vi "流量计.vi"() -> ()   [LabVIEW 2016, in "流量计集成.lvlib"]
uses:
  <vilib>/Plasmionique/MB Master/MB_Master_Serial/MB_Master_Serial.lvclass
  D:/Program Files (x86)/National Instruments/LabVIEW 2016/vi.lib/Plasmionique/MB Master/MB_Master/MB_Master.lvclass
  <vilib>/Analysis/baseanly.llb/Mean (DBL).vi
  <vilib>/Utility/config.llb/NI_LVConfig.lvlib
  <vilib>/Analysis/NI_AALBase.lvlib
panel:
  in  "运行模式":enum16{"按周期模式", "全常规模式"}(ring)=enum."全常规模式"
  in  "流量计启用 5":bool
  in  "数量 5":u16
  out "流量计类型 5":T1=enum."WL1A1明渠流量计"
  in  "流量计启用 4":bool
  in  "数量 4":u16
  out "流量计类型 4":T1=enum."博意达流量计"
  out "平均水位":dbl
  out "总累积流量":dbl
  out "平均流速":dbl
  out "总流量":dbl
  in  "选项卡控件":T2(tab)
  out "数组":T3[](array[typedef])
  out "数组 2":T4[](array[typedef]) {"累积流量单位" items=["L", "M3", "T", "USG"]; "瞬时流量单位" items=["L/S", "L/M", "L/H", "M3/S", "M3/M", "M3/H", "T/S", "T/M", "T/H", "GPS", "GPM", "GPH"]}
  out "数组 3":T7[](array[typedef])
  out "数组 4":T3[](array[typedef])
  out "数组 5":T3[](array[typedef])
  out "MB_Serial session":refnum<class "MB_Master_Serial.lvclass">
  in  "斯坦道功率测流":bool
  in  "流量计启用 3":bool
  in  "数量 3":u16
  out "流量计类型 3":T1=enum."斯坦道功率测流"
  in  "流量计启用 2":bool
  in  "数量 2":u16
  out "流量计类型 2":T1=enum."MGG/KL QC"
  in  "数量":u16
  out "流量计类型":T1
  in  "流量计启用":bool
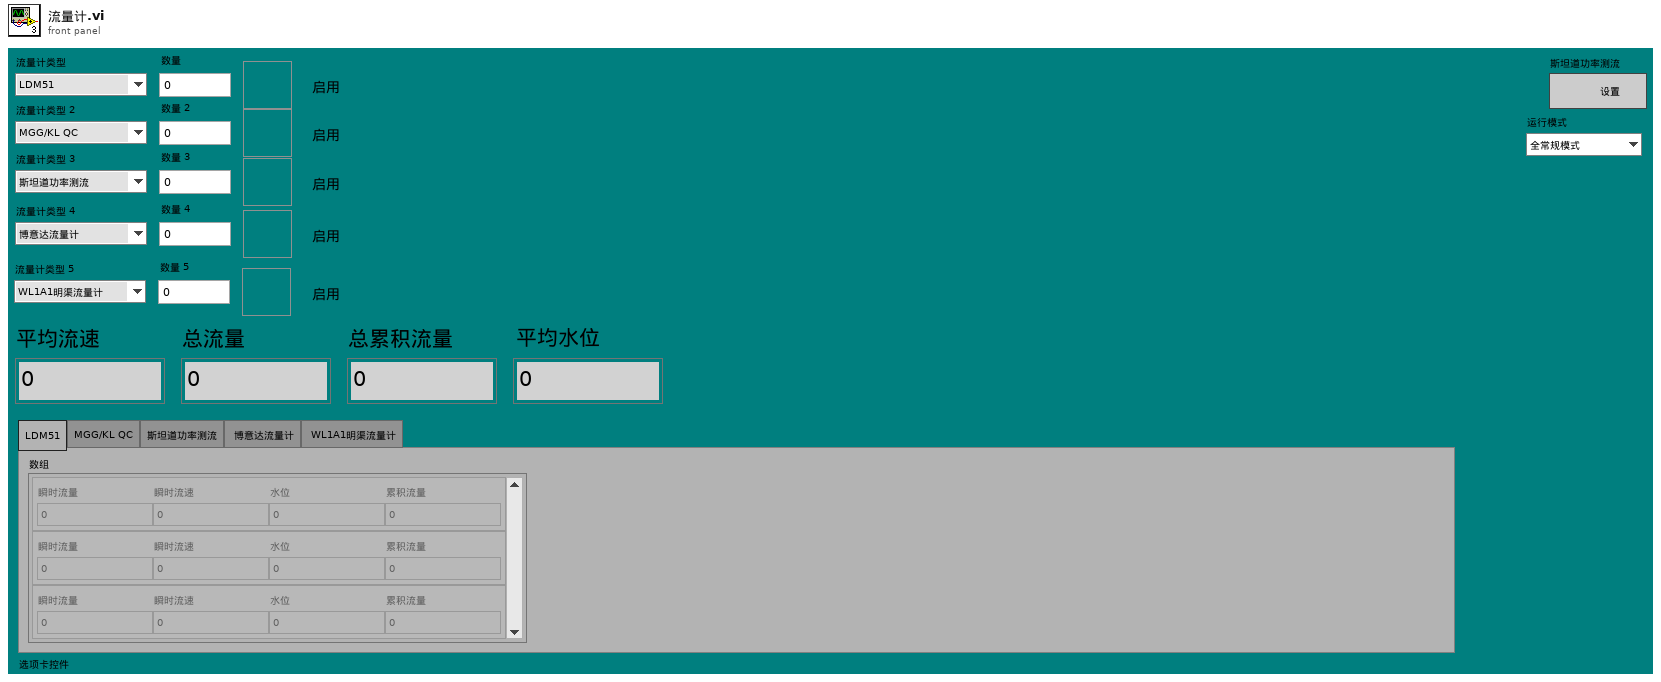
[diagram p1: front panel]
types:
  T1 = typedef "流量计集成.lvlib/流量计类型.ctl" = enum16{"LDM51", "MGG/KL QC", "斯坦道功率测流", "博意达流量计", "SL1500-3G", "WL1A1明渠流量计"}
  T2 = enum32{"LDM51", "MGG/KL QC", "斯坦道功率测流", " 博意达流量计", " WL1A1明渠流量计"}
  T3 = typedef "流量计集成.lvlib/LDM51明渠流量计.lvlib/读取值.ctl" = cluster{"瞬时流量":sgl, "瞬时流速":sgl, "水位":sgl, "累积流量":sgl}
  T4 = typedef "流量计集成.lvlib/MGG-KL-QC流量计.lvlib/读取值.ctl" = cluster{"瞬时流量":sgl, "瞬时流速":sgl, "流量百分比":sgl, "流体电导比":sgl, "正向累积数值":sgl, "反向累积数值":sgl, "瞬时流量单位":T5, "累积流量单位":T6, "上限报警":u16, "下限报警":u16, "空管报警":u16, "系统报警":u16}
  T5 = typedef "流量计集成.lvlib/MGG-KL-QC流量计.lvlib/瞬时流量单位.ctl" = u16
  T6 = typedef "流量计集成.lvlib/MGG-KL-QC流量计.lvlib/累积流量单位.ctl" = u16
  T7 = typedef "流量计集成.lvlib/斯坦道功率测流.lvlib/状态值.ctl" = cluster{"1号瞬时流量":dbl, "2号瞬时流量":dbl, "3号瞬时流量":dbl, "4号瞬时流量":dbl, "5号瞬时流量":dbl, "6号瞬时流量":dbl, "1号累积流量":dbl, "2号累积流量":dbl, "3号累积流量":dbl, "4号累积流量":dbl, "5号累积流量":dbl, "6号累积流量":dbl, "总瞬时流量":dbl, "总累积流量":dbl}
  T8 = cluster{"时间标识":timestamp, "测量模式":string, "数据类型":string, "监测值":sgl, "单位":string, "数据标识":string, "因子编码":string}
  T9 = typedef "LVDateTimeRec.ctl" = cluster{"秒数的小数部分":dbl, "秒":i32, "分":i32, "时":i32, "日":i32, "月":i32, "年":i32, "天数（周）":i32, "天数（年）":i32, "DST":i32}
  T10 = typedef "流量计集成.lvlib/博意达流量计.lvlib/读取值.ctl" = cluster{"瞬时流量":sgl, "瞬时流速":sgl, "水位":sgl, "累积流量":sgl}
  T11 = typedef "NI_LVConfig.lvlib/Config Data RefNum.ctl" = refnum<k1>
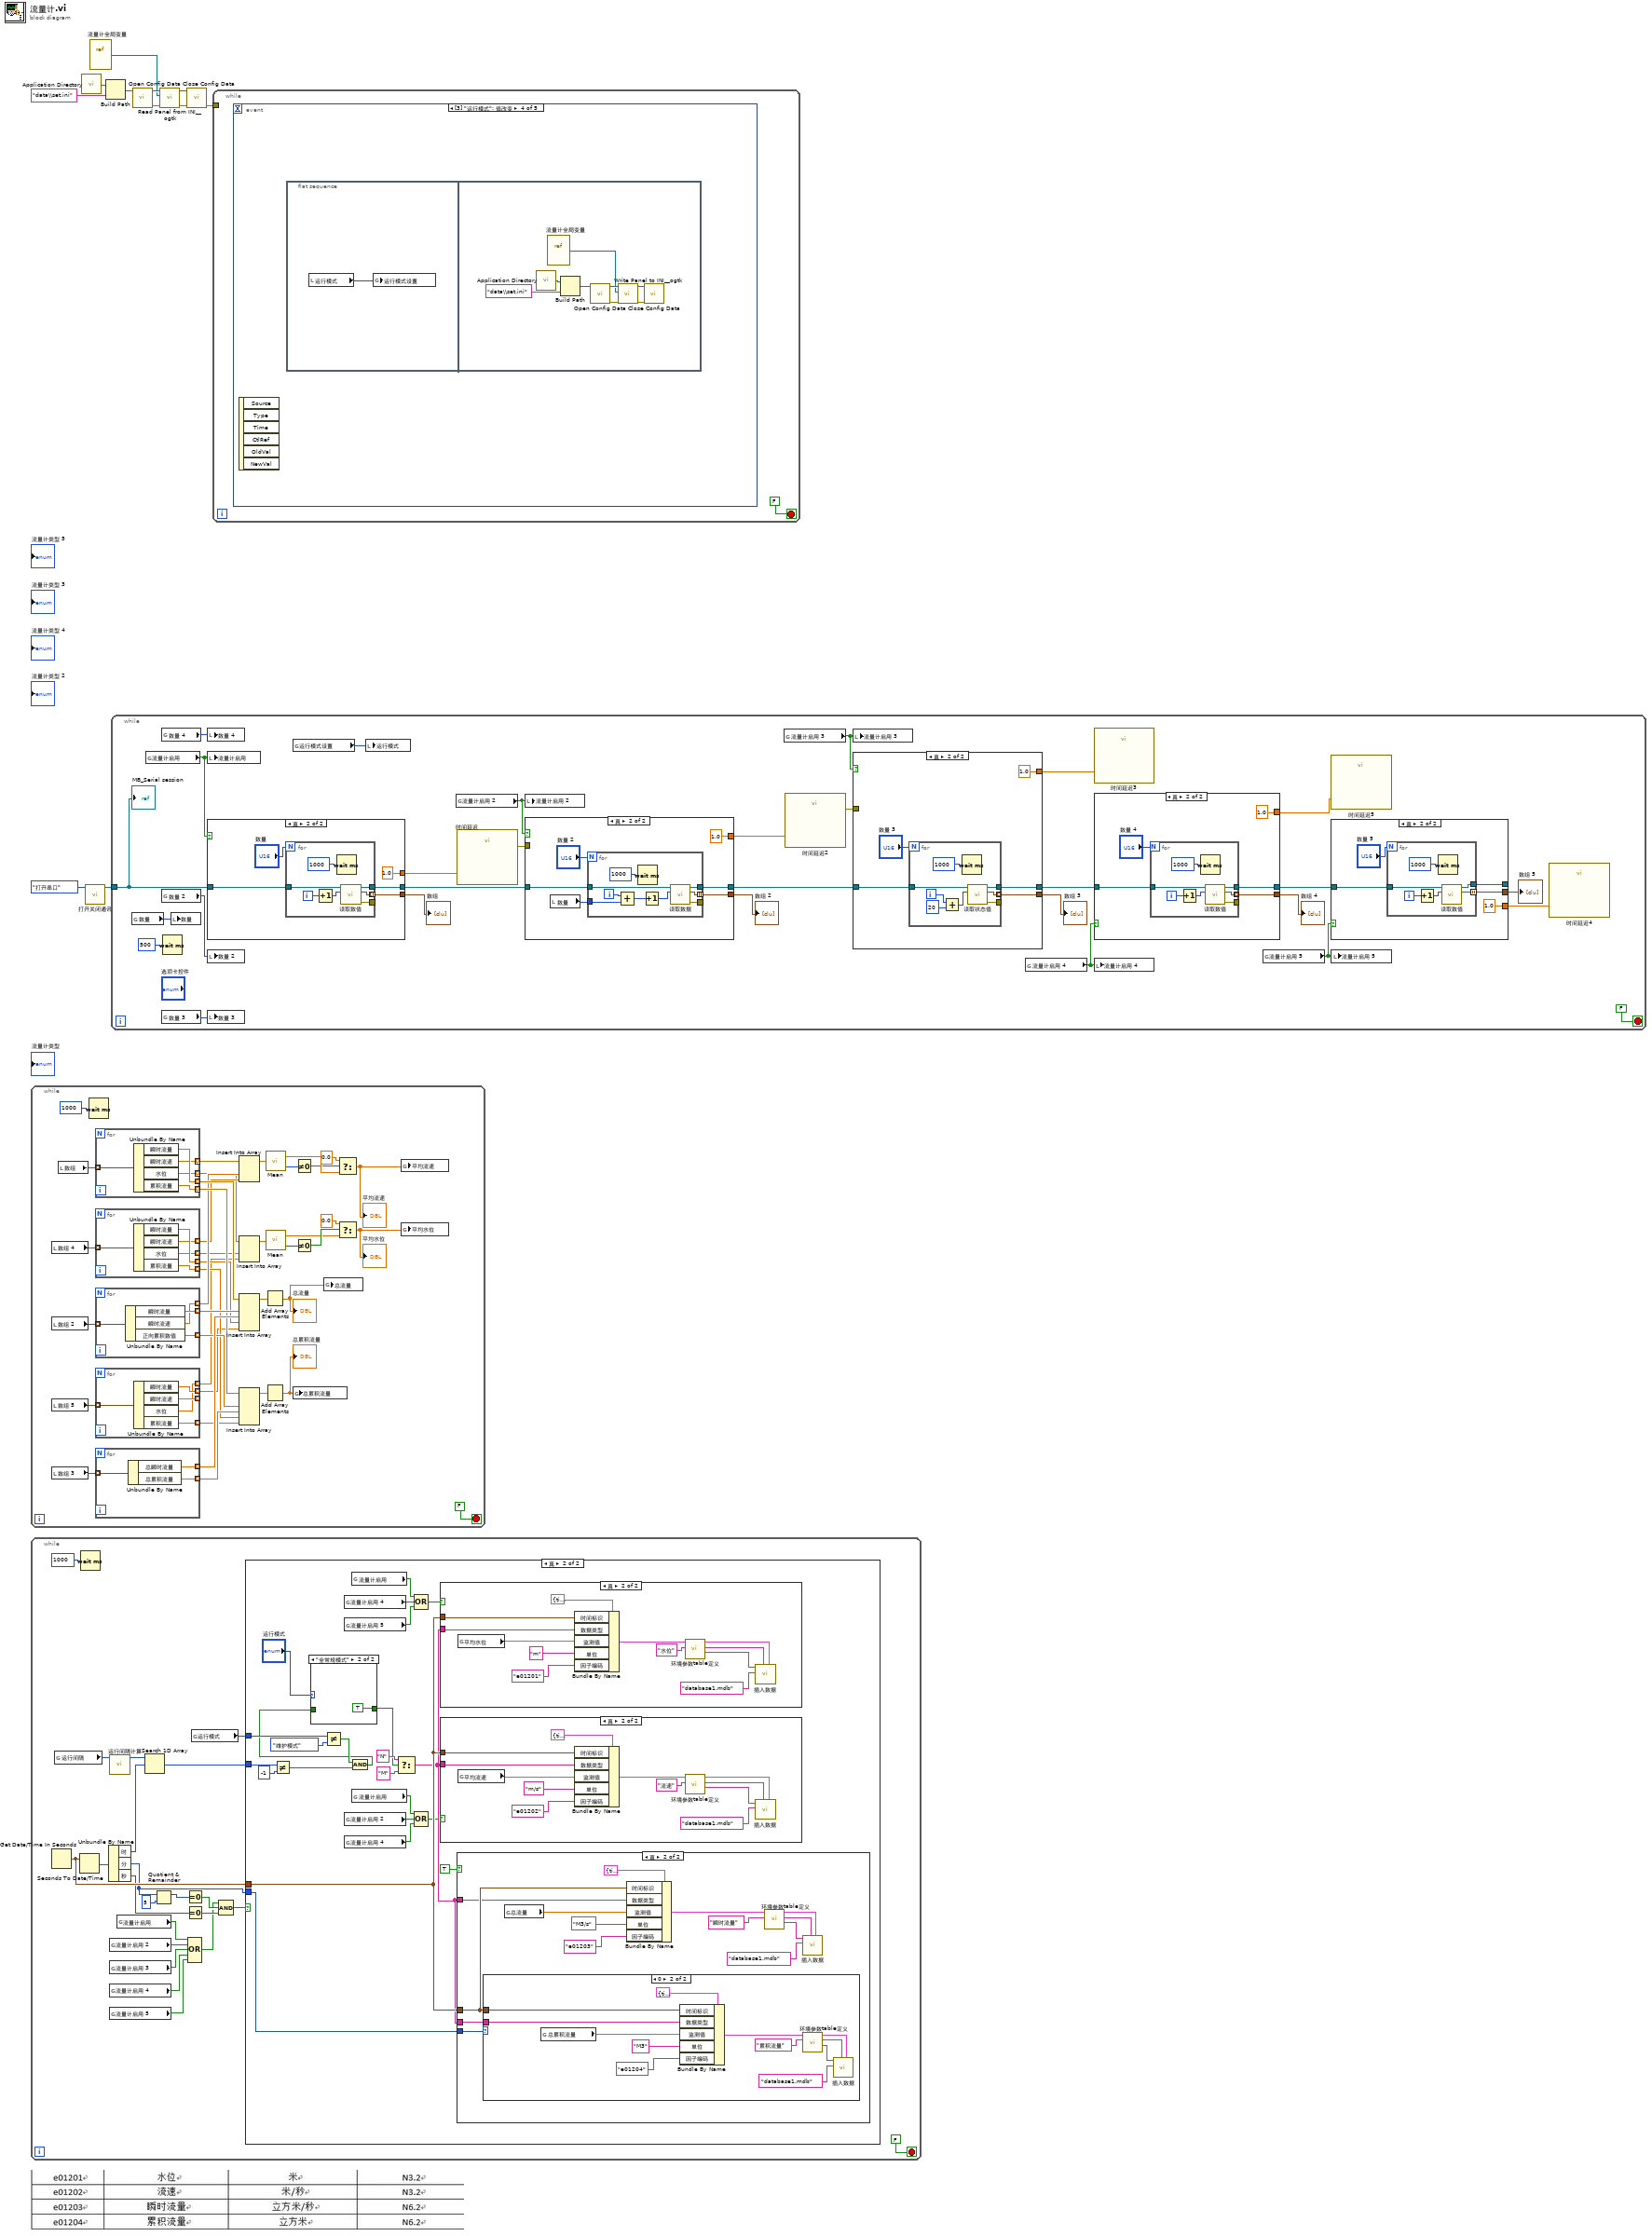
[diagram p0: block diagram]
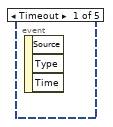
[diagram p8: hidden frame]
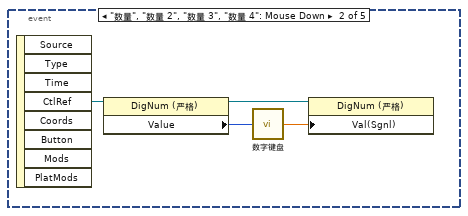
[diagram p9: hidden frame]
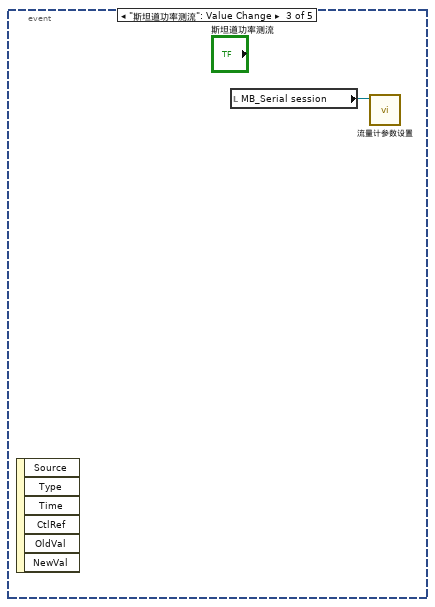
[diagram p10: hidden frame]
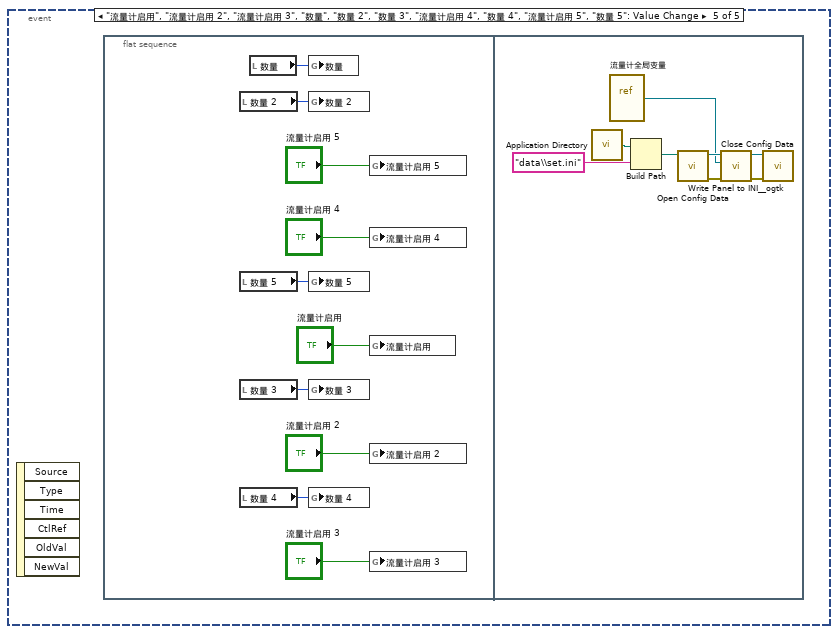
[diagram p11: hidden frame]
diagram:
  n1 = while {
    stop <- FALSE stop-if-true
    n2 = local read "数组 4"() -> (w22:T3[])
    n3 = local read "数组 2"() -> (w47:T4[])
    n4 = local read "数组 5"() -> (w15:T3[])
    n5 = local read "数组 3"() -> (w46:T7[])
    n6 = local read "数组"() -> (w50:T3[])
    n7 = Wait (ms)(milliseconds to wait=u32 1000 ("等待时间（毫秒）")) -> ()  [unwired: 1 out]
    n8 = for {
      tunnel: w50 -> [w72] mode=indexing
      tunnel: [w71] -> w45 mode=indexing
      tunnel: [w70] -> w37 mode=indexing
      tunnel: [w69] -> w19 mode=indexing
      tunnel: [w68] -> w42 mode=indexing
      n9 = Unbundle By Name(w72) -> ("瞬时流量"=w71:sgl, "瞬时流速"=w70:sgl, "水位"=w69:sgl, "累积流量"=w68:sgl)
    }
    n10 = for {
      tunnel: w22 -> [w60] mode=indexing
      tunnel: [w59] -> w20 mode=indexing
      tunnel: [w58] -> w21 mode=indexing
      tunnel: [w57] -> w17 mode=indexing
      tunnel: [w56] -> w16 mode=indexing
      n11 = Unbundle By Name(w60) -> ("瞬时流量"=w59:sgl, "瞬时流速"=w58:sgl, "水位"=w57:sgl, "累积流量"=w56:sgl)
    }
    n12 = for {
      tunnel: w47 -> [w67] mode=indexing
      tunnel: [w66] -> w44 mode=indexing
      tunnel: [w65] -> w36 mode=indexing
      tunnel: [w64] -> w41 mode=indexing
      n13 = Unbundle By Name(w67) -> ("瞬时流量"=w66:sgl, "瞬时流速"=w65:sgl, "正向累积数值"=w64:sgl)
    }
    n14 = for {
      tunnel: w15 -> [w55] mode=indexing
      tunnel: [w54] -> w13 mode=indexing
      tunnel: [w53] -> _ mode=indexing
      tunnel: [w52] -> w12 mode=indexing
      tunnel: [w51] -> w14 mode=indexing
      n15 = Unbundle By Name(w55) -> ("瞬时流量"=w54:sgl, "瞬时流速"=w53:sgl, "水位"=w52:sgl, "累积流量"=w51:sgl)
    }
    n16 = for {
      tunnel: w46 -> [w63] mode=indexing
      tunnel: [w62] -> w43 mode=indexing
      tunnel: [w61] -> w40 mode=indexing
      n17 = Unbundle By Name(w63) -> ("总瞬时流量"=w62:dbl, "总累积流量"=w61:dbl)
    }
    n18 = Insert Into Array(array=w37, new element #1=w36, new element #2=w21) -> (w31:sgl[])  [unwired: 1 in]
    n19 = Insert Into Array(array=w19, new element #1=w17, new element #2=w12) -> (w18:sgl[])  [unwired: 1 in]
    n20 = Insert Into Array(array=w45, new element #1=w44, new element #2=w43, new element #3=w20, new element #4=w13) -> (w39:sgl[])  [unwired: 1 in]
    n21 = Insert Into Array(array=w42, new element #1=w41, new element #2=w40, new element #3=w16, new element #4=w14) -> (w38:sgl[])  [unwired: 1 in]
    n22 = Add Array Elements(numeric array=w39) -> (sum=w26:sgl)
    "总流量" <- w26
    n23 = Add Array Elements(numeric array=w38) -> (sum=w24:sgl)
    "总累积流量" <- w24
    n24 = call-poly <vilib>:"Mean.vi"("X"=w31) -> ("mean"=w35:dbl, "error"=w32:i32)
    n25 = call-poly <vilib>:"Mean.vi"("X"=w18) -> ("mean"=w27:dbl, "error"=w30:i32)
    n26 = global write "流量计全局变量.vi" "总累积流量"(w24) -> ()
    n27 = Not Equal To 0?(x=w32) -> (x != 0?=w33:bool)
    n28 = Not Equal To 0?(x=w30) -> (x != 0?=w29:bool)
    n29 = global write "流量计全局变量.vi" "总流量"(w26) -> ()
    n30 = Select(t=0.0, s=w33, f=w35) -> (s? t:f=w25:dbl)
    "平均流速" <- w25
    n31 = Select(t=0.0, s=w29, f=w27) -> (s? t:f=w23:dbl)
    "平均水位" <- w23
    n32 = global write "流量计全局变量.vi" "平均流速"(w25) -> ()
    n33 = global write "流量计全局变量.vi" "平均水位"(w23) -> ()
  }
  n34 = while {
    stop <- FALSE stop-if-true
    n35 = Get Date/Time In Seconds() -> (seconds since 1Jan1904=w93:timestamp)
    n36 = global read "流量计全局变量.vi" "运行间隔"() -> (w76:i16)
    n37 = Seconds To Date/Time(time stamp (now)=w93) -> (date time rec=w92:T9)  [unwired: 1 in]
    n38 = Wait (ms)(milliseconds to wait=u32 1000 ("等待时间（毫秒）")) -> ()  [unwired: 1 out]
    n39 = Unbundle By Name(w92) -> ("时"=w80:i32, "分"=w77:i32, "秒"=w90:i32)
    n40 = global read "流量计全局变量.vi" "流量计启用 2"() -> (w83:bool)
    n41 = global read "流量计全局变量.vi" "流量计启用 3"() -> (w82:bool)
    n42 = global read "流量计全局变量.vi" "流量计启用 4"() -> (w75:bool)
    n43 = global read "流量计全局变量.vi" "流量计启用 5"() -> (w74:bool)
    n44 = call "运行间隔计算.vi"("运行周期"=w76) -> ("数组"=w79:i32[])  [unwired: 10 in]
    n45 = global read "流量计全局变量.vi" "流量计启用"() -> (w84:bool)
    n46 = Search 1D Array(1D array=w79, element=w80) -> (index of element=w78:i32)  [unwired: 1 in]
    n47 = Quotient & Remainder(x=w77, y=5) -> (x-y*floor(x/y)=w89:i32)  [unwired: 1 out]
    n48 = Equal To 0?(x=w89) -> (x = 0?=w88:bool)
    n49 = Equal To 0?(x=w90) -> (x = 0?=w87:bool)
    n50 = Compound Arithmetic op=OR ("复合运算")(w84, w83, w82, w75, w74) -> (w81:bool)
    n51 = global read "流量计全局变量.vi" "运行模式"() -> (w73:enum16{"维护模式", "常规模式", "应急模式", "质控模式"})
    n52 = Compound Arithmetic op=AND ("复合运算")(w81, w88, w87) -> (w86:bool)
    n53 = case shown="真" w86 {
      tunnel: w93 -> [_ w117]
      tunnel: w78 -> [_ w110]
      tunnel: w77 -> [_ w109]
      tunnel: w73 -> [_ w100]
      frame False {
      }
      frame True {
        n54 = Not Equal?(x=w110, y=-1) -> (x != y?=w113:bool)
        n55 = Not Equal?(x=w100, y=enum16{"维护模式", "常规模式", "应急模式", "质控模式"}."维护模式") -> (x != y?=w98:bool)
        n56 = global read "流量计全局变量.vi" "流量计启用 4"() -> (w103:bool)
        n57 = global read "流量计全局变量.vi" "流量计启用 5"() -> (w102:bool)
        n58 = global read "流量计全局变量.vi" "流量计启用 2"() -> (w115:bool)
        n59 = global read "流量计全局变量.vi" "流量计启用 4"() -> (w107:bool)
        n60 = And(x=w98, y=w113) -> (x .and. y?=w96:bool)
        n61 = case shown="\"全常规模式\"" "运行模式" {
          tunnel: w96 -> [w118 _]
          tunnel: [w118 TRUE] -> w95
          frame "按周期模式", Default {
          }
          frame "全常规模式" {
          }
        }
        n62 = global read "流量计全局变量.vi" "流量计启用"() -> (w104:bool)
        n63 = global read "流量计全局变量.vi" "流量计启用"() -> (w116:bool)
        n64 = Select(t="N" ("单位"), s=w95, f="M" ("单位")) -> (s? t:f=w108:string)
        n65 = Compound Arithmetic op=OR ("复合运算")(w104, w103, w102) -> (w101:bool)
        n66 = Compound Arithmetic op=OR ("复合运算")(w116, w115, w107) -> (w105:bool)
        n67 = case shown="真" w101 {
          tunnel: w117 -> [_ w127]
          tunnel: w108 -> [_ w126]
          frame False {
          }
          frame True {
            n68 = global read "流量计全局变量.vi" "平均水位"() -> (w125:dbl)
            n69 = Bundle By Name(cluster=T8 {"时间标识"=timestamp(0 s since 1904-01-01), "测量模式"="水样测试", "数据类型"="N", "监测值"=0.0, "单位"="mg/L", "数据标识"="N", "因子编码"=""} ("data"), "时间标识"=w127, "数据类型"=w126, "监测值"=w125, "单位"="m", "因子编码"="e01201") -> (w121:T8)
            n70 = call "环境参数table定义.vi"("table 输入"="水位", "data"=w121) -> ("table 输出"=w122:string, "columns"=w123:string[], "data输出"=w124:T8)  [unwired: 7 in]
            n71 = call "插入数据.vi"("data"=w124, "columns"=w123, "database"="database1.mdb" ("table 输入"), "table"=w122) -> ()  [unwired: 7 in, 1 out]
          }
        }
        n72 = case shown="真" w105 {
          tunnel: w117 -> [_ w164]
          tunnel: w108 -> [_ w163]
          frame False {
          }
          frame True {
            n73 = global read "流量计全局变量.vi" "平均流速"() -> (w165:dbl)
            n74 = Bundle By Name(cluster=T8 {"时间标识"=timestamp(0 s since 1904-01-01), "测量模式"="水样测试", "数据类型"="N", "监测值"=0.0, "单位"="mg/L", "数据标识"="N", "因子编码"=""} ("data"), "时间标识"=w164, "数据类型"=w163, "监测值"=w165, "单位"="m/s", "因子编码"="e01202") -> (w161:T8)
            n75 = call "环境参数table定义.vi"("table 输入"="流速", "data"=w161) -> ("table 输出"=w158:string, "columns"=w159:string[], "data输出"=w160:T8)  [unwired: 7 in]
            n76 = call "插入数据.vi"("data"=w160, "columns"=w159, "database"="database1.mdb" ("table 输入"), "table"=w158) -> ()  [unwired: 7 in, 1 out]
          }
        }
        n77 = case shown="真" TRUE {
          tunnel: w117 -> [_ w140]
          tunnel: w108 -> [_ w144]
          tunnel: w109 -> [_ w143]
          tunnel: w108 -> [_ w138]
          frame False {
          }
          frame True {
            n78 = case shown="0" w143 {
              tunnel: w140 -> [_ w156]
              tunnel: w144 -> [_ w153]
              frame Default {
              }
              frame 0 {
                n79 = global read "流量计全局变量.vi" "总累积流量"() -> (w154:dbl)
                n80 = Bundle By Name(cluster=T8 {"时间标识"=timestamp(0 s since 1904-01-01), "测量模式"="水样测试", "数据类型"="N", "监测值"=0.0, "单位"="mg/L", "数据标识"="N", "因子编码"=""} ("data"), "时间标识"=w156, "数据类型"=w153, "监测值"=w154, "单位"="M3", "因子编码"="e01204") -> (w150:T8)
                n81 = call "环境参数table定义.vi"("table 输入"="累积流量", "data"=w150) -> ("table 输出"=w146:string, "columns"=w147:string[], "data输出"=w148:T8)  [unwired: 7 in]
                n82 = call "插入数据.vi"("data"=w148, "columns"=w147, "database"="database1.mdb" ("table 输入"), "table"=w146) -> ()  [unwired: 7 in, 1 out]
              }
            }
            n83 = global read "流量计全局变量.vi" "总流量"() -> (w139:dbl)
            n84 = Bundle By Name(cluster=T8 {"时间标识"=timestamp(0 s since 1904-01-01), "测量模式"="水样测试", "数据类型"="N", "监测值"=0.0, "单位"="mg/L", "数据标识"="N", "因子编码"=""} ("data"), "时间标识"=w140, "数据类型"=w138, "监测值"=w139, "单位"="M3/s", "因子编码"="e01203") -> (w136:T8)
            n85 = call "环境参数table定义.vi"("table 输入"="瞬时流量", "data"=w136) -> ("table 输出"=w132:string, "columns"=w133:string[], "data输出"=w134:T8)  [unwired: 7 in]
            n86 = call "插入数据.vi"("data"=w134, "columns"=w133, "database"="database1.mdb" ("table 输入"), "table"=w132) -> ()  [unwired: 7 in, 1 out]
          }
        }
      }
    }
  }
  n87 = call <vilib>:"Application Directory.vi"() -> ("Application Directory"=w9:path)
  n88 = call "打开关闭通讯.vi"("功能输入"=enum16{"打开串口", "关闭串口"}."打开串口") -> ("MB_Serial session"=w1:refnum<class "MB_Master_Serial.lvclass">)  [unwired: 9 in, 1 out]
  n89 = vi-ref "流量计全局变量.vi"() -> (w3:refnum<vi>)
  n90 = Build Path(base path=w9, name or relative path="data\\set.ini" ("名称或相对路径")) -> (appended path=w10:path)
  n91 = while {
    tunnel: w1 -> [w188]
    stop <- FALSE stop-if-true
    n92 = global read "流量计全局变量.vi" "数量"() -> (w187:u16)
    n93 = global read "流量计全局变量.vi" "流量计启用"() -> (w196:bool)
    n94 = global read "流量计全局变量.vi" "数量 4"() -> (w175:u16)
    n95 = global read "流量计全局变量.vi" "数量 2"() -> (w186:u16)
    n96 = global read "流量计全局变量.vi" "数量 3"() -> (w185:u16)
    n97 = Wait (ms)(milliseconds to wait=u32 500 ("等待时间（毫秒）")) -> ()  [unwired: 1 out]
    n98 = local write "数量"(w187) -> ()
    n99 = local write "数量 4"(w175) -> ()
    n100 = local write "流量计启用"(w196) -> ()
    n101 = case shown="真" w196 {
      tunnel: w188 -> [w254 w259]
      tunnel: [w254 w257] -> w195
      tunnel: [_ w256] -> w193
      tunnel: [_ 1.0 ("Delay Time (s)")] -> w184
      frame False {
      }
      frame True {
        n102 = for {
          N: "数量" -> [_]
          tunnel: w259 -> [w266]
          tunnel: [w265] -> _
          tunnel: [w262] -> w257
          tunnel: [w261] -> w256 mode=indexing
          i -> [w264]
          n103 = Increment(x=w264) -> (x+1=w263:i32)
          n104 = Wait (ms)(milliseconds to wait=u32 1000 ("等待时间（毫秒）")) -> ()  [unwired: 1 out]
          n105 = call "读取数值.vi"("Slave ID"=w263, "MB session in"=w266) -> ("error out"=w265:errorcluster, "读取值"=w261:T3, "MB session out"=w262:refnum<class "MB_Master_Serial.lvclass">)  [unwired: 7 in]
        }
      }
    }
    "数组" <- w193
    n106 = local write "数量 2"(w186) -> ()
    n107 = local write "数量 3"(w185) -> ()
    n108 = global read "流量计全局变量.vi" "运行模式设置"() -> (w170:enum16{"按周期模式", "全常规模式"})
    n109 = local write "运行模式"(w170) -> ()
    n110 = global read "流量计全局变量.vi" "流量计启用 2"() -> (w194:bool)
    n111 = call "时间延迟"("Delay Time (s)"=w184) -> ("error out"=w183:errorcluster)  [unwired: 10 in]
    n112 = local write "流量计启用 2"(w194) -> ()
    n113 = case shown="真" w194 {
      tunnel: w195 -> [w238 w243]
      tunnel: [w238 w241] -> w191
      tunnel: [_ w240] -> w192
      tunnel: w183 -> [_ _]
      tunnel: [_ 1.0 ("Delay Time (s)")] -> w182
      frame False {
      }
      frame True {
        n114 = local read "数量"() -> (w242:u16)
        n115 = for {
          N: "数量 2" -> [_]
          tunnel: w243 -> [w252]
          tunnel: w242 -> [w249]
          tunnel: [w248] -> w241
          tunnel: [w247] -> w240 mode=indexing
          tunnel: [w246] -> _
          i -> [w250]
          n116 = Add(x=w250, y=w249) -> (x+y=w251:i32)
          n117 = Wait (ms)(milliseconds to wait=u32 1000 ("等待时间（毫秒）")) -> ()  [unwired: 1 out]
          n118 = Increment(x=w251) -> (x+1=w253:i32)
          n119 = call "读取数据.vi"("Slave ID"=w253, "MB session in"=w252) -> ("error out"=w246:errorcluster, "读取值"=w247:T4, "MB session out"=w248:refnum<class "MB_Master_Serial.lvclass">)  [unwired: 6 in, 1 out]
        }
      }
    }
    "数组 2" <- w192
    n120 = global read "流量计全局变量.vi" "流量计启用 3"() -> (w190:bool)
    n121 = call "时间延迟2"("Delay Time (s)"=w182) -> ("error out"=w180:errorcluster)  [unwired: 10 in]
    n122 = local write "流量计启用 3"(w190) -> ()
    n123 = case shown="真" w190 {
      tunnel: w191 -> [w224 w229]
      tunnel: [w224 w228] -> w177
      tunnel: [_ w226] -> w189
      tunnel: [_ 1.0 ("Delay Time (s)")] -> w181
      tunnel: w180 -> [_ _]
      frame False {
      }
      frame True {
        n124 = for {
          N: "数量 3" -> [_]
          tunnel: w229 -> [w235]
          tunnel: [w232] -> w228
          tunnel: [w233] -> _
          tunnel: [w231] -> w226 mode=indexing
          i -> [w237]
          n125 = Add(x=w237, y=20) -> (x+y=w234:i32)
          n126 = Wait (ms)(milliseconds to wait=u32 1000 ("等待时间（毫秒）")) -> ()  [unwired: 1 out]
          n127 = call "读取状态值.vi"("Slave ID"=w234, "MB session in"=w235) -> ("error out"=w233:errorcluster, "状态值"=w231:T7, "MB session out"=w232:refnum<class "MB_Master_Serial.lvclass">)  [unwired: 6 in, 1 out]
        }
      }
    }
    "数组 3" <- w189
    n128 = global read "流量计全局变量.vi" "流量计启用 4"() -> (w178:bool)
    n129 = call "时间延迟3"("Delay Time (s)"=w181) -> ()  [unwired: 10 in, 1 out]
    n130 = case shown="真" w178 {
      tunnel: w177 -> [w211 w216]
      tunnel: [w211 w215] -> w171
      tunnel: [_ w214] -> w176
      tunnel: [_ 1.0 ("Delay Time (s)")] -> w179
      frame False {
      }
      frame True {
        n131 = for {
          N: "数量 4" -> [_]
          tunnel: w216 -> [w223]
          tunnel: [w221] -> w215
          tunnel: [w222] -> _
          tunnel: [w220] -> w214 mode=indexing
          i -> [w218]
          n132 = Increment(x=w218) -> (x+1=w217:i32)
          n133 = Wait (ms)(milliseconds to wait=u32 1000 ("等待时间（毫秒）")) -> ()  [unwired: 1 out]
          n134 = call "读取数值.vi"("Slave ID"=w217, "MB session in"=w223) -> ("error out"=w222:errorcluster, "读取值"=w220:T10, "MB session out"=w221:refnum<class "MB_Master_Serial.lvclass">)  [unwired: 7 in]
        }
      }
    }
    "数组 4" <- w176
    n135 = local write "流量计启用 4"(w178) -> ()
    n136 = global read "流量计全局变量.vi" "流量计启用 5"() -> (w173:bool)
    n137 = call "时间延迟5"("Delay Time (s)"=w179) -> ()  [unwired: 10 in, 1 out]
    n138 = case shown="真" w173 {
      tunnel: w171 -> [w199 w204]
      tunnel: [w199 w203] -> _
      tunnel: [_ w202] -> w174
      tunnel: [_ 1.0 ("Delay Time (s)")] -> w172
      frame False {
      }
      frame True {
        n139 = for {
          N: "数量 5" -> [_]
          tunnel: w204 -> [w207]
          tunnel: [w205] -> w203
          tunnel: [w206] -> w202 mode=indexing
          i -> [w209]
          n140 = Increment(x=w209) -> (x+1=w208:i32)
          n141 = Wait (ms)(milliseconds to wait=u32 1000 ("等待时间（毫秒）")) -> ()  [unwired: 1 out]
          n142 = call "读取数值.vi"("Slave ID"=w208, "MB session in"=w207) -> ("读取值"=w206:T10, "MB session out"=w205:refnum<class "MB_Master_Serial.lvclass">)  [unwired: 7 in, 1 out]
        }
      }
    }
    "数组 5" <- w174
    n143 = local write "流量计启用 5"(w173) -> ()
    n144 = call "时间延迟4"("Delay Time (s)"=w172) -> ()  [unwired: 10 in, 1 out]
    "MB_Serial session" <- w188
  }
  n145 = call <vilib>:"Open Config Data.vi"("configuration file path"=w10) -> ("error out"=w7:errorcluster, "refnum"=w8:T11)  [unwired: 8 in, 1 out]
  n146 = call <userlib>:"Read Panel from INI__ogtk.vi"("error in (no error)"=w7, "VI ref"=w3, "refnum"=w8) -> ("error out"=w5:errorcluster, "refnum out"=w6:T11)  [unwired: 7 in]
  n147 = call <vilib>:"Close Config Data.vi"("error in (no error)"=w5, "refnum"=w6) -> ("error out"=w4:errorcluster)  [unwired: 8 in, 1 out]
  n148 = while {
    tunnel: w4 -> [_]
    stop <- FALSE stop-if-true
    n149 = event shown="[3] \"运行模式\": 值改变" {
      selector: _ -> [_ _ _ _ _]
      dyn-events: _ -> [_ _ _ _ _]
      timeout: _ -> [_ _ _ _ _]
      event Timeout {
        n150 = event-data() -> ()  [unwired: 1 in, 3 out]
      }
      event "数量", "数量 2", "数量 3", "数量 4": Mouse Down {
        n151 = event-data() -> ("CtlRef"=w271:refnum<vi>)  [unwired: 1 in, 7 out]
        n152 = property class="DigNum (严格)"(reference=w271) -> (reference out=w269:refnum<vi>, "Value"=w270:u16)  [unwired: 1 in, 1 out]
        n153 = call "数字键盘.vi"("OldNumber"=w270) -> ("NewNumber"=w268:dbl)
        n154 = property class="DigNum (严格)"(reference=w269, "Val(Sgnl)"=w268) -> ()  [unwired: 1 in, 2 out]
      }
      event "斯坦道功率测流": Value Change {
        n155 = event-data() -> ()  [unwired: 1 in, 6 out]
        n156 = local read "MB_Serial session"() -> (w272:refnum<class "MB_Master_Serial.lvclass">)
        n157 = call "流量计参数设置.vi"("MB session in"=w272) -> ()  [unwired: 11 in]
      }
      event "运行模式": Value Change {
        n158 = event-data() -> ()  [unwired: 1 in, 6 out]
        n159 = flat-sequence {
          frame #0 {
            n160 = local read "运行模式"() -> (w273:enum16{"按周期模式", "全常规模式"})
            n161 = global write "流量计全局变量.vi" "运行模式设置"(w273) -> ()
          }
          frame #1 {
            n162 = call <vilib>:"Application Directory.vi"() -> ("Application Directory"=w277:path)
            n163 = vi-ref "流量计全局变量.vi"() -> (w274:refnum<vi>)
            n164 = Build Path(base path=w277, name or relative path="data\\set.ini" ("名称或相对路径")) -> (appended path=w276:path)
            n165 = call <vilib>:"Open Config Data.vi"("configuration file path"=w276) -> ("error out"=w279:errorcluster, "refnum"=w281:T11)  [unwired: 8 in, 1 out]
            n166 = call <userlib>:"Write Panel to INI__ogtk.vi"("error in (no error)"=w279, "VI ref"=w274, "refnum"=w281) -> ("error out"=w278:errorcluster, "refnum out"=w280:T11)  [unwired: 7 in]
            n167 = call <vilib>:"Close Config Data.vi"("error in (no error)"=w278, "refnum"=w280) -> ()  [unwired: 8 in, 2 out]
          }
        }
      }
      event "流量计启用", "流量计启用 2", "流量计启用 3", "数量", "数量 2", "数量 3", "流量计启用 4", "数量 4", "流量计启用 5", "数量 5": Value Change {
        n168 = event-data() -> ()  [unwired: 1 in, 6 out]
        n169 = flat-sequence {
          frame #0 {
            n170 = local read "数量 2"() -> (w287:u16)
            n171 = local read "数量 5"() -> (w282:u16)
            n172 = local read "数量 3"() -> (w286:u16)
            n173 = local read "数量 4"() -> (w284:u16)
            n174 = local read "数量"() -> (w288:u16)
            n175 = global write "流量计全局变量.vi" "数量"(w288) -> ()
            n176 = global write "流量计全局变量.vi" "数量 2"(w287) -> ()
            n177 = global write "流量计全局变量.vi" "数量 5"(w282) -> ()
            n178 = global write "流量计全局变量.vi" "数量 3"(w286) -> ()
            n179 = global write "流量计全局变量.vi" "数量 4"(w284) -> ()
            n180 = global write "流量计全局变量.vi" "流量计启用 5"("流量计启用 5") -> ()
            n181 = global write "流量计全局变量.vi" "流量计启用 4"("流量计启用 4") -> ()
            n182 = global write "流量计全局变量.vi" "流量计启用"("流量计启用") -> ()
            n183 = global write "流量计全局变量.vi" "流量计启用 2"("流量计启用 2") -> ()
            n184 = global write "流量计全局变量.vi" "流量计启用 3"("流量计启用 3") -> ()
          }
          frame #1 {
            n185 = call <vilib>:"Application Directory.vi"() -> ("Application Directory"=w295:path)
            n186 = vi-ref "流量计全局变量.vi"() -> (w292:refnum<vi>)
            n187 = Build Path(base path=w295, name or relative path="data\\set.ini" ("名称或相对路径")) -> (appended path=w294:path)
            n188 = call <vilib>:"Open Config Data.vi"("configuration file path"=w294) -> ("error out"=w297:errorcluster, "refnum"=w299:T11)  [unwired: 8 in, 1 out]
            n189 = call <userlib>:"Write Panel to INI__ogtk.vi"("error in (no error)"=w297, "VI ref"=w292, "refnum"=w299) -> ("error out"=w296:errorcluster, "refnum out"=w298:T11)  [unwired: 7 in]
            n190 = call <vilib>:"Close Config Data.vi"("error in (no error)"=w296, "refnum"=w298) -> ()  [unwired: 8 in, 2 out]
          }
        }
      }
    }
  }
